vi "Waveform - Get Time Array.vi"() -> ()   [LabVIEW 2020]
doc: "Shows how to use the Get Waveform Time Array VI."
uses:
  <vilib>/Waveform/WDTOps.llb/WDT Get Waveform Time Array DBL.vi
panel:
  in  "dt":dbl=0.01 min=0.0 step=0.01
  out "X Array Timestamps (s)":dbl[](array[numeric])
  # "Overview: Demonstrates how to retrieve an array of timestamps from a waveform with the Get Waveform Time Array VI.\nInstructions:\n1. Specify a dt value.\n2. Run the VI. Any array of numeric values representing the timestamps of each data point in the simulated waveform will be displayed in the X Array Timestamps indicator."
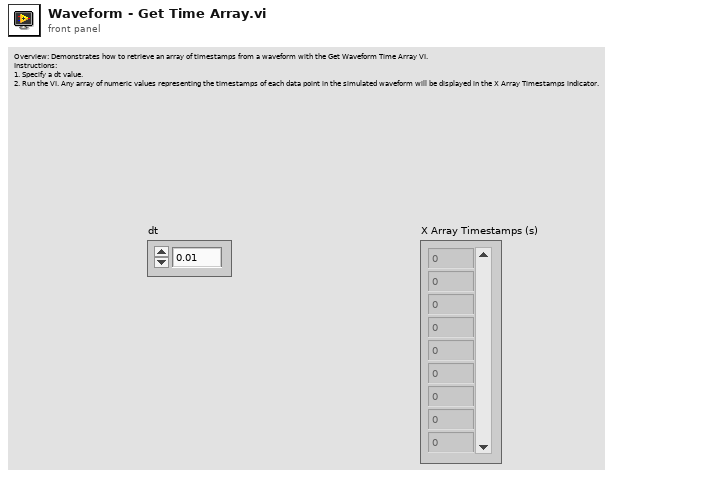
[diagram p1: front panel]
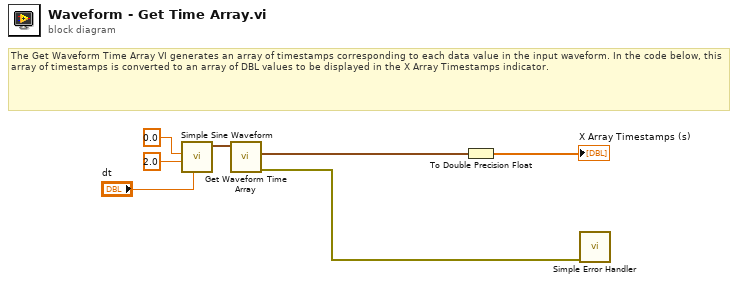
[diagram p0: block diagram]
diagram:
  # "The Get Waveform Time Array VI generates an array of timestamps corresponding to each data value in the input waveform. In the code below, this array of timestamps is converted to an array of DBL values to be displayed in the X Array Timestamps indicator."
  n1 = call "Simple Sine Waveform.vi"("delta t"="dt", "n cycles"=2.0 ("frequency"), "t0"=0.0) -> ("sine waveform"=w7:waveform(dbl))  [unwired: 8 in]
  n2 = call-poly <vilib>:"Get Waveform Time Array.vi"("waveform in"=w7) -> ("error out"=w4:errorcluster, "X array"=w3:timestamp[])  [unwired: 9 in]
  n3 = To Double Precision Float(number=w3) -> (double precision float=→"X Array Timestamps (s)":dbl[])
  n4 = call <vilib>:"Simple Error Handler.vi"("error in (no error)"=w4) -> ()  [unwired: 4 in, 5 out]
